vi "Get Outgoing Cyclic Signals.vi"(7 "Name":string, 8 "error in":errorcluster, 9 "Mermory Table Offset":u32, 10 "database in":refnum<k21>, 11 "Item Ref":T7 format="%.0x") -> (0 "error out":errorcluster, 1 "Outgoing Cyclic Configuraiton":T1 {"Outgoing Cyclic Frame"."Transmit Propreties"."Transmit Time" format="%#_p"; "Channel Pairs"."Block Data Refs"."Data Reference" format="%.0x"}, 3 "Item Ref out":T7 format="%.0x")   [LabVIEW 2015, in "J1939 Addon System Explorer.lvlib"]
uses:
  J1939 Addon System Explorer.lvlib
  <vilib>/NI Veristand/Custom Device API/Custom Device Item Ref.ctl
  Shared/Types/SysDef Outgoing Cyclic Configurations.ctl
  Shared/Types/SysDef Outgoing Frame Configuration.ctl
  Shared/Types/XNET Frame Event Properties.ctl
  Shared/Types/Outgoing Cyclic Channel Pairs.ctl
  <vilib>/NI Veristand/Custom Device API/Block Data Reference.ctl
  <vilib>/NI Veristand/Custom Device API/Data Reference.ctl
  <vilib>/NI Veristand/Custom Device API/Data Access Type.ctl
  <vilib>/NI Veristand/Custom Device API/Get Item Property (Variant).vi
  <vilib>/NI Veristand/Custom Device API/Get Item Property (U32).vi
  <vilib>/NI Veristand/Custom Device Tools/Custom Device Utility Library/NI VeriStand - Search for All Items by GUID.vi
  Shared/SubVIs/Constants.vi
  Shared/J1939 Addon Shared.lvlib
  <vilib>/NI VeriStand/Custom Device API/Custom Device API.lvlib
  <vilib>/NI Veristand/Custom Device Tools/Custom Device Utility Library/Custom Device Utility Library.lvlib
  <resource>/objmgr/xnet.rc
panel:
  out "database out":refnum<k21>
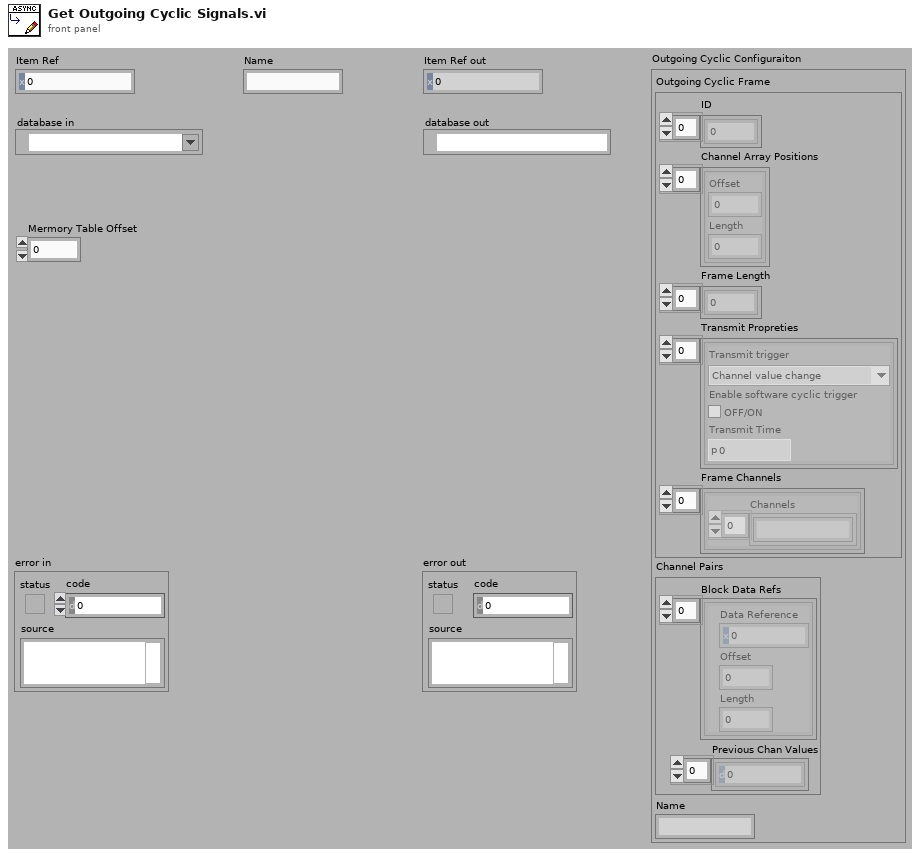
[diagram p1: front panel]
types:
  T1 = typedef "J1939 Addon Shared.lvlib/SysDef Outgoing Cyclic Configurations.ctl" = cluster{"Outgoing Cyclic Frame":T2, "Channel Pairs":T4, "Name":string}
  T2 = typedef "J1939 Addon Shared.lvlib/SysDef Outgoing Frame Configuration.ctl" = cluster{"ID":u32[], "Channel Array Positions":cluster{"Offset":u32, "Length":u32}[], "Frame Length":u32[], "Transmit Propreties":T3[], "Frame Channels":cluster{"Channels":string[]}[]}
  T3 = typedef "J1939 Addon Shared.lvlib/XNET Frame Event Properties.ctl" = cluster{"Transmit trigger":enum16{"Channel value change"}, "Enable software cyclic trigger":bool, "Transmit Time":dbl}
  T4 = typedef "J1939 Addon Shared.lvlib/Outgoing Cyclic Channel Pairs.ctl" = cluster{"Block Data Refs":T5[], "Previous Chan Values":dbl[]}
  T5 = typedef "Custom Device API.lvlib/Block Data Reference.ctl" = cluster{"Data Reference":T6, "Offset":u64, "Length":u64}
  T6 = typedef "Custom Device API.lvlib/Data Reference.ctl" = i32
  T7 = typedef "Custom Device API.lvlib/Custom Device Item Ref.ctl" = u64
  T8 = typedef "Custom Device API.lvlib/Data Access Type.ctl" = enum16{"Read", "Write"}
  T9 = typedef "Custom Device API.lvlib/Custom Device Item Info.ctl" = cluster{"Name":string, "Is Channel":bool, "GUID":string, "Is Waveform":bool}
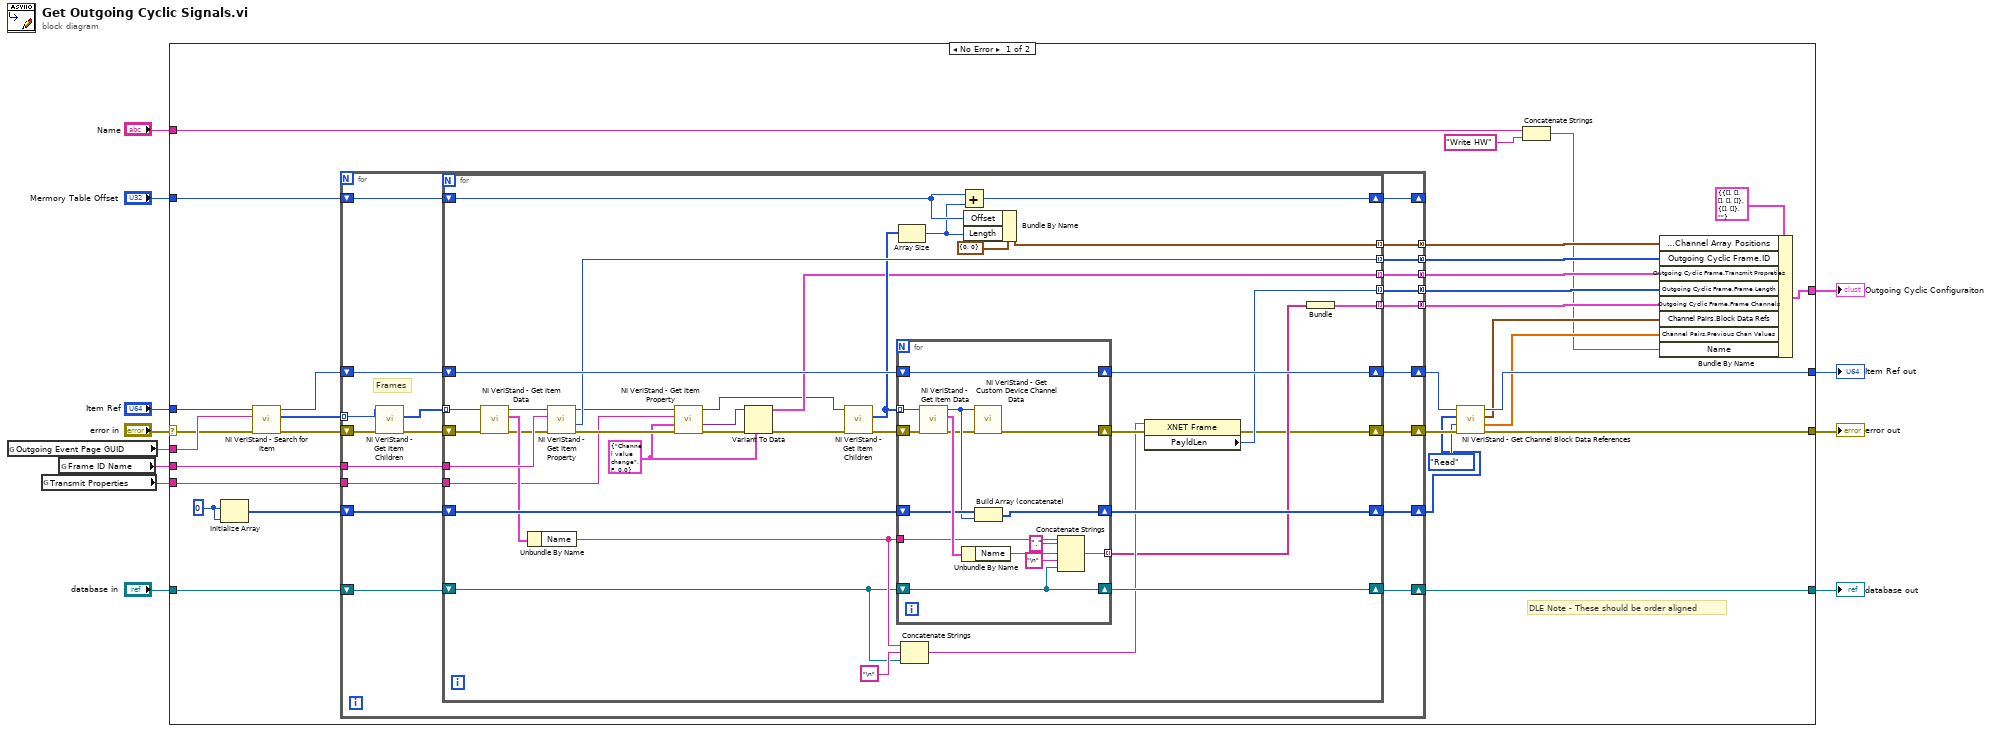
[diagram p0: block diagram]
diagram:
  n1 = global read "Constants.vi" "Outgoing Event Page GUID"() -> (w7:string)
  n2 = global read "Constants.vi" "Transmit Properties"() -> (w3:string)
  n3 = global read "Constants.vi" "Frame ID Name"() -> (w10:string)
  n4 = case shown="No Error" "error in" {
    selector: "error in" -> [w14 w117]
    tunnel: "database in" -> [w37 w118]
    tunnel: [w31 w116] -> w11
    tunnel: [w40 _] -> w4
    tunnel: w10 -> [w43 _]
    tunnel: [w19 w117] -> w9
    tunnel: "Item Ref" -> [w13 w116]
    tunnel: w7 -> [w42 _]
    tunnel: [w41 w118] -> w6
    tunnel: w3 -> [w35 _]
    tunnel: "Mermory Table Offset" -> [w27 _]
    tunnel: "Name" -> [w21 _]
    frame No Error {
      w29 = T7 0 ("Item Ref out")
      # "DLE Note - These should be order aligned"
      n5 = Initialize Array(w29, w29) -> (w28:T7[])
      n6 = call-poly <vilib>:"NI VeriStand - Search for Item.vi"("error in"=w14, "Item GUID"=w42, "Section Ref in"=w13) -> ("error out"=w17:errorcluster, "Item Refs"=w15:T7[], "Section Ref out"=w16:T7)  [unwired: 5 in, 1 out]
      n7 = for {
        tunnel: w43 -> [w63]
        tunnel: [w60] -> w39 mode=concatenating
        tunnel: [w59] -> w38 mode=concatenating
        tunnel: [w56] -> w36 mode=concatenating
        tunnel: w35 -> [w55]
        tunnel: [w54] -> w34 mode=concatenating
        tunnel: [w50] -> w26 mode=concatenating
        shift-right: [w61] -> w41
        shift-left: w37 -> [w58]
        shift-right: [w49] -> w25
        shift-left: w28 -> [w52]
        shift-right: [w48] -> w24
        shift-left: w16 -> [w46]
        shift-right: [w45] -> _
        shift-left: w27 -> [w51]
        shift-right: [w53] -> w33
        shift-left: w17 -> [w47]
        tunnel: w15 -> [w44] mode=indexing
        # "Frames"
        n8 = call <vilib>:"NI VeriStand - Get Item Children.vi"("error in (no error)"=w47, "Item Ref in"=w44) -> ("error out"=w57:errorcluster, "Child Refs"=w62:T7[])  [unwired: 6 in, 2 out]
        n9 = for {
          shift-right: [w64] -> w53
          shift-left: w57 -> [w85]
          tunnel: w62 -> [w86] mode=indexing
          tunnel: w63 -> [w100]
          shift-right: [w99] -> w61
          shift-left: w58 -> [w78]
          shift-right: [w96] -> w48
          shift-left: w46 -> [w97]
          shift-right: [w94] -> w49
          shift-left: w52 -> [w95]
          tunnel: [w65] -> w60 mode=indexing
          tunnel: [w93] -> w50 mode=indexing
          shift-right: [w91] -> w45
          shift-left: w51 -> [w89]
          tunnel: [w87] -> w59 mode=indexing
          tunnel: [w83] -> w56 mode=indexing
          tunnel: w55 -> [w73]
          tunnel: [w68] -> w54 mode=indexing
          w70 = T3 {"Transmit trigger"=enum."Channel value change", "Enable software cyclic trigger"=FALSE, "Transmit Time"=0.0} ("Cluster")
          n10 = call <vilib>:"NI VeriStand - Get Item Data.vi"("error in (no error)"=w85, "Item Ref in"=w86) -> ("error out"=w81:errorcluster, "Item Info"=w84:T9, "Item Ref out"=w82:T7)  [unwired: 6 in, 1 out]
          n11 = Unbundle By Name(w84) -> ("Name"=w79:string)
          n12 = call-poly <vilib>:"NI VeriStand - Get Item Property.vi"("error in (no error)"=w81, "Property Name"=w100, "Item Ref in"=w82) -> ("error out"=w75:errorcluster, "Value"=w93:u32, "Item Ref out"=w74:T7)  [unwired: 5 in, 1 out]
          n13 = call-poly <vilib>:"NI VeriStand - Get Item Property.vi"("error in (no error)"=w75, "Default Value"=w70, "Property Name"=w73, "Item Ref in"=w74) -> ("error out"=w72:errorcluster, "Value"=w69:variant, "Item Ref out"=w67:T7)  [unwired: 4 in, 1 out]
          n14 = Variant To Data(error in=w72, type=w70, Variant=w69) -> (data=w68:T3, error out=w71:errorcluster)
          n15 = call <vilib>:"NI VeriStand - Get Item Children.vi"("error in (no error)"=w71, "Item Ref in"=w67) -> ("error out"=w98:errorcluster, "Child Refs"=w92:T7[])  [unwired: 6 in, 2 out]
          n16 = for {
            shift-right: [w101] -> w77
            shift-left: w98 -> [w114]
            tunnel: w92 -> [w115] mode=indexing
            tunnel: [w110] -> w66 mode=indexing
            shift-right: [w109] -> w99
            shift-left: w78 -> [w109]
            shift-right: [w104] -> w96
            shift-left: w97 -> [w104]
            shift-right: [w107] -> w94
            shift-left: w95 -> [w108]
            tunnel: w79 -> [w106]
            n17 = call <vilib>:"NI VeriStand - Get Item Data.vi"("error in (no error)"=w114, "Item Ref in"=w115) -> ("error out"=w102:errorcluster, "Item Info"=w113:T9, "Item Ref out"=w103:T7)  [unwired: 6 in, 1 out]
            n18 = Unbundle By Name(w113) -> ("Name"=w112:string)
            n19 = call <vilib>:"NI VeriStand - Get Custom Device Channel Data.vi"("error in (no error)"=w102, "Channel Ref in"=w103) -> ("error out"=w101:errorcluster)  [unwired: 4 in, 5 out]
            n20 = Build Array (concatenate)(w108, w103) -> (w107:T7[])
            n21 = Concatenate Strings(w106, "." ("string"), w112, "\n" ("string"), w109) -> (w110:string)
          }
          n22 = Array Size(array=w92) -> (size(s)=w88:i32)
          n23 = Concatenate Strings(w79, "\n" ("string"), w78) -> (w76:string)
          n24 = Add(x=w89, y=w88) -> (x+y=w91:u32)
          n25 = Bundle By Name(cluster=cluster{"Offset":u32, "Length":u32} {"Offset"=0, "Length"=0} ("Channel Array Position"), "Offset"=w89, "Length"=w88) -> (w87:cluster{"Offset":u32, "Length":u32})
          n26 = property class="XNET Frame"(reference=w76, error in=w77) -> (error out=w64:errorcluster, "PayldLen"=w83:u32)  [unwired: 1 out]
          n27 = Bundle(w66) -> (w65:cluster{string[]})  [unwired: 1 in]
        }
      }
      n28 = call <vilib>:"NI VeriStand - Get Channel Block Data References.vi"("error in (no error)"=w33, "Access"=Data_Access_Type."Read", "Channel Refs"=w25, "Device Ref in"=w24) -> ("error out"=w19:errorcluster, "Values Array"=w22:dbl[], "Block Data Refs"=w23:T5[], "Device Ref out"=w31:T7)  [unwired: 4 in]
      n29 = Concatenate Strings(w21, "Write HW" ("name (unnamed)")) -> (w18:string)
      n30 = Bundle By Name(cluster=T1 {"Outgoing Cyclic Frame"={"ID"=[], "Channel Array Positions"=[], "Frame Length"=[], "Transmit Propreties"=[], "Frame Channels"=[]}, "Channel Pairs"={"Block Data Refs"=[], "Previous Chan Values"=[]}, "Name"=""} ("Outgoing Cyclic Configuraiton"), "Outgoing Cyclic Frame.Channel Array Positions"=w38, "Outgoing Cyclic Frame.ID"=w26, "Outgoing Cyclic Frame.Transmit Propreties"=w34, "Outgoing Cyclic Frame.Frame Length"=w36, "Outgoing Cyclic Frame.Frame Channels"=w39, "Channel Pairs.Block Data Refs"=w23, "Channel Pairs.Previous Chan Values"=w22, "Name"=w18) -> (w40:T1)
    }
    frame Error {
    }
  }
  "error out" <- w9
  "database out" <- w6
  "Item Ref out" <- w11
  "Outgoing Cyclic Configuraiton" <- w4
